vi "LogErrorEvent(Caller).vi"(8 "Error In":errorcluster) -> (0 "Error Out":errorcluster)   [LabVIEW 2019, in "EventLogger.lvlib"]
uses:
  EventLogger.lvlib
  Enum - Message.ctl
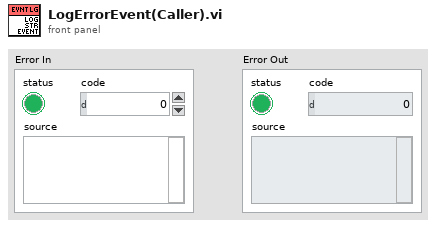
[diagram p1: front panel]
types:
  T1 = typedef "EventLogger.lvlib/Enum - Message.ctl" = enum16{"Initialize", "Idle", "CreateLog", "LogStrEvent", "LogErrorEvent", "LogVICall", "Error", "Exit"}
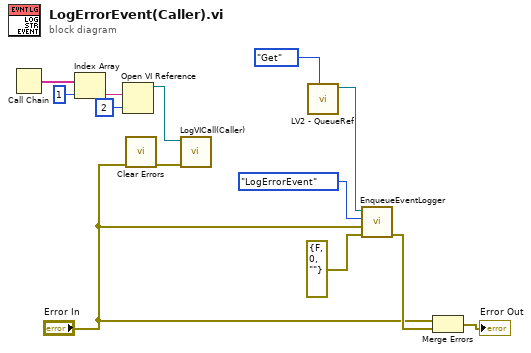
[diagram p0: block diagram]
diagram:
  n1 = Call Chain() -> (call chain=w9:string[])
  n2 = Index Array(array=w9, index=1) -> (element=w7:string)
  n3 = Open VI Reference(vi path=w7, options=2) -> (vi reference=w5:refnum<vi>)  [unwired: 4 in, 1 out]
  n4 = call <vilib>:"Clear Errors.vi"("error in (no error)"="Error In") -> ("error out"=w4:errorcluster)  [unwired: 5 in, 1 out]
  n5 = call "LogVICall(Caller).vi"("Error In"=w4, "Caller VI"=w5) -> ()  [unwired: 9 in, 1 out]
  n6 = call "LV2 - QueueRef.vi"("Action"=enum16{"Set", "Get"}."Get") -> ("EventLoggerQueue out"=w11:refnum<queue>)  [unwired: 10 in]
  n7 = call "EnqueueEventLogger.vi"("Error In"=errorcluster {"status"=FALSE, "code"=0, "source"=""}, "Data"="Error In", "Message"=Enum_-_Message."LogErrorEvent", "EventLoggerQueue"=w11) -> ("Error Out"=w12:errorcluster)  [unwired: 6 in, 1 out]
  n8 = Merge Errors("Error In", w12) -> (→"Error Out":errorcluster)
